vi "addNode.vi"(0 "reference":refnum<class "PackageNode.lvclass">, 1 "node":refnum<class "AbstractNode.lvclass">, 2 "point2D":T1 {"y" format="%.2f"; "x" format="%.2f"}, 5 "error in (no error)":errorcluster) -> (14 "reference out":refnum<class "PackageNode.lvclass">, 15 "added":bool, 19 "error out":errorcluster)   [LabVIEW 2016, in "PackageNode.lvclass"]
doc: "public boolean addNode(Node n, Point2D p)"
uses:
  <resource>/Framework/Providers/Open_GDS/UML/PackageNode_class/PackageNode.lvclass
  C:/Program Files (x86)/National Instruments/LabVIEW 2016/resource/Framework/Providers/Open_GDS/UML/AbstractNode_class/AbstractNode.lvclass
  <resource>/Framework/Providers/Open_GDS/UML/AbstractNode_class/AbstractNode.lvclass
  <resource>/Framework/Providers/Open_GDS/UML/General/Point/Point Point2D.ctl
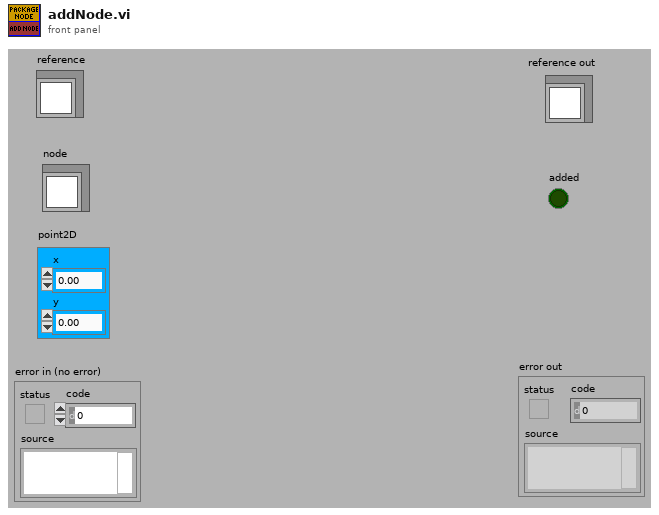
[diagram p1: front panel]
types:
  T1 = typedef "Point Point2D.ctl" = cluster{"x":dbl, "y":dbl}
  T2 = typedef "PackageNode.lvclass/ObjectAttributes.ctl" = cluster{"name":string, "contents":refnum<class "MultiLineString.lvclass">, "DEFAULT_TOP_WIDTH":i32, "DEFAULT_TOP_HEIGHT":i32, "DEFAULT_WIDTH":i32, "DEFAULT_HEIGHT":i32, "NAME_GAP":i32, "XGAP":i32, "YGAP":i32, "Collapsed":bool, "Note color":u32, "Justification":u16}
  T3 = typedef "AbstractNode.lvclass/ObjectAttributes.ctl" = cluster{"parent":refnum<class "AbstractNode.lvclass">, "children":refnum<class "AbstractNode.lvclass">[], "Hidden":bool}
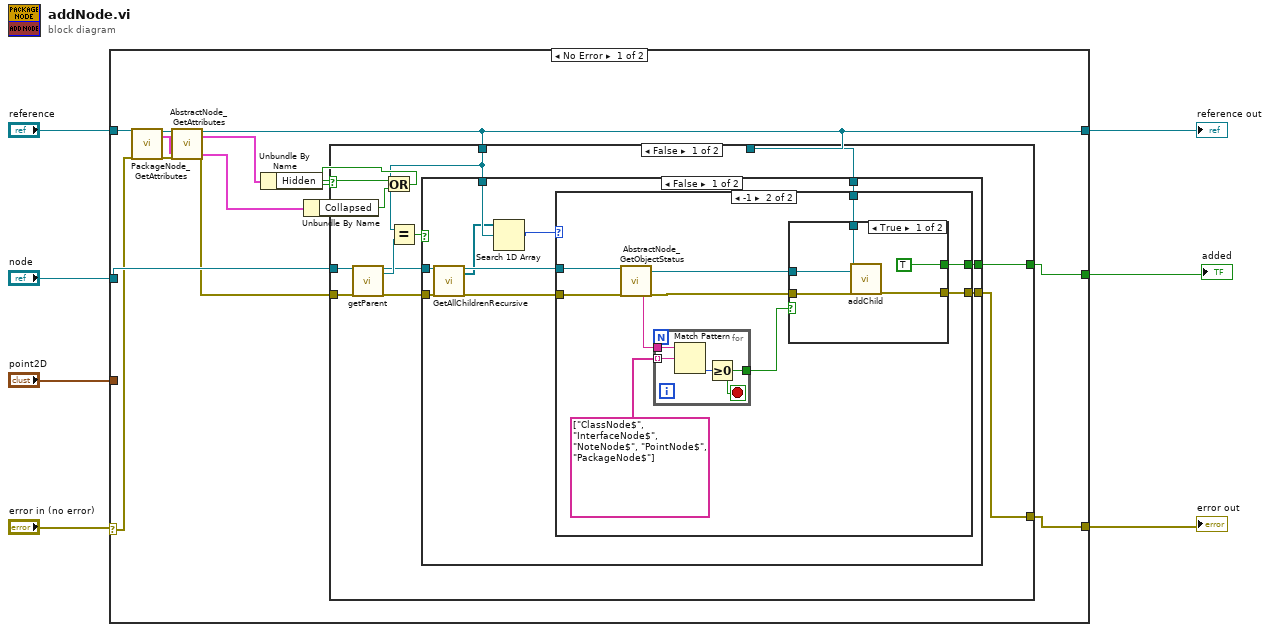
[diagram p0: block diagram]
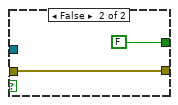
[diagram p3: hidden frame]
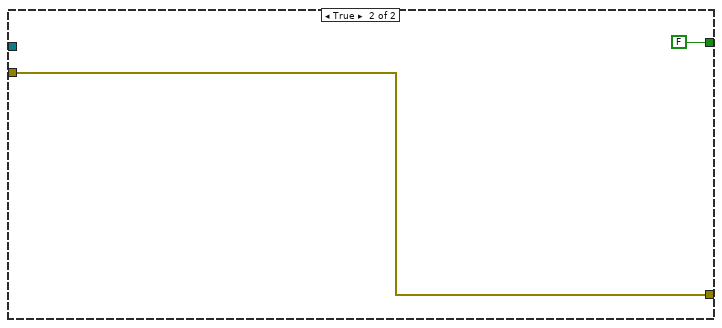
[diagram p5: hidden frame]
diagram:
  n1 = case shown="No Error" "error in (no error)" {
    selector: "error in (no error)" -> [w17 w67]
    tunnel: "reference" -> [w18 w68]
    tunnel: [w21 w67] -> w6
    tunnel: [w9 w68] -> w5
    tunnel: "node" -> [w20 _]
    tunnel: "point2D" -> [_ _]
    tunnel: [w19 _] -> w1
    frame No Error {
      n2 = call <resource>:"PackageNode_GetAttributes.vi"("reference in"=w18, "error in (no error)"=w17) -> ("reference out"=w12:refnum<class "PackageNode.lvclass">, "Data"=w13:T2, "error out"=w11:errorcluster)  [unwired: 14 in, 1 out]
      n3 = call <resource>:"AbstractNode_GetAttributes.vi"("reference in"=w12, "error in (no error)"=w11) -> ("reference out"=w9:refnum<class "PackageNode.lvclass">, "Data"=w8:T3, "error out"=w10:errorcluster)  [unwired: 14 in, 1 out]
      n4 = Unbundle By Name(w8) -> ("Hidden"=w16:bool)
      n5 = Unbundle By Name(w13) -> ("Collapsed"=w15:bool)
      n6 = Or(x=w16, y=w15) -> (x .or. y?=w14:bool)
      n7 = case shown="False" w14 {
        tunnel: [w31 w65] -> w21
        tunnel: w20 -> [w28 _]
        tunnel: [w30 FALSE] -> w19
        tunnel: w9 -> [w29 _]
        tunnel: w10 -> [w27 w65]
        tunnel: w9 -> [w24 _]
        frame False {
          n8 = call-dynamic "getParent.vi"("reference"=w28, "error in (no error)"=w27) -> ("reference out"=w22:refnum<class "AbstractNode.lvclass">, "parentNode"=w25:refnum<class "AbstractNode.lvclass">, "error out"=w26:errorcluster)  [unwired: 13 in, 2 out]
          n9 = Equal?(x=w24, y=w25) -> (x = y?=w23:bool)
          n10 = case shown="False" w23 {
            tunnel: [w41 w64] -> w31
            tunnel: [w40 _] -> w30
            tunnel: w29 -> [w39 _]
            tunnel: w24 -> [w36 _]
            tunnel: w26 -> [w33 w64]
            tunnel: w22 -> [w32 _]
            frame False {
              n11 = call <resource>:"GetAllChildrenRecursive.vi"("reference"=w32, "error in (no error)"=w33) -> ("reference out"=w38:refnum<class "AbstractNode.lvclass">, "children"=w35:refnum<class "AbstractNode.lvclass">[], "error out"=w37:errorcluster)  [unwired: 15 in]
              n12 = Search 1D Array(1D array=w35, element=w36) -> (index of element=w34:i32)  [unwired: 1 in]
              n13 = case shown="-1" w34 {
                tunnel: [w42 w52] -> w41
                tunnel: [_ w51] -> w40
                tunnel: w39 -> [_ w47]
                tunnel: w38 -> [_ w46]
                tunnel: w37 -> [w42 w45]
                frame 0, Default {
                }
                frame -1 {
                  n14 = call <resource>:"AbstractNode_GetObjectStatus.vi"("reference in"=w46, "error in (no error)"=w45) -> ("Class name"=w43:string, "reference out"=w49:refnum<class "AbstractNode.lvclass">, "error out"=w50:errorcluster)  [unwired: 15 out]
                  n15 = for {
                    tunnel: w43 -> [w63]
                    tunnel: string[] ["ClassNode$", "InterfaceNode$", "NoteNode$", "PointNode$", "PackageNode$"] -> [w62] mode=indexing
                    tunnel: [w60] -> w44
                    stop <- w60 stop-if-true
                    n16 = Match Pattern(string=w63, regular expression=w62) -> (offset past match=w61:i32)  [unwired: 4 out]
                    n17 = Greater Or Equal To 0?(x=w61) -> (x >= 0?=w60:bool)
                  }
                  n18 = case shown="True" w44 {
                    tunnel: [TRUE FALSE] -> w51
                    tunnel: w50 -> [w56 w59]
                    tunnel: [w53 w59] -> w52
                    tunnel: w47 -> [w55 _]
                    tunnel: w49 -> [w54 _]
                    frame True {
                      n19 = call-dynamic "addChild.vi"("reference"=w55, "node"=w54, "error in (no error)"=w56) -> ("error out"=w53:errorcluster)  [unwired: 15 in, 1 out]
                    }
                    frame False {
                    }
                  }
                }
              }
            }
            frame True {
            }
          }
        }
        frame True {
        }
      }
    }
    frame Error {
    }
  }
  "reference out" <- w5
  "error out" <- w6
  "added" <- w1
